vi "Read ModuleA Configuration.vi"(8 "error in (no error)":errorcluster, 11 "ModuleA in":refnum<class "System.lvclass">) -> (0 "error out":errorcluster, 2 "Configuration":T1, 3 "ModuleA out":refnum<class "System.lvclass">)   [LabVIEW 2014, in "System.lvclass"]
uses:
  System.lvclass
  Configuration - cluster.ctl
  <vilib>/JKI/JKI SMO/SMO/SMO.lvclass
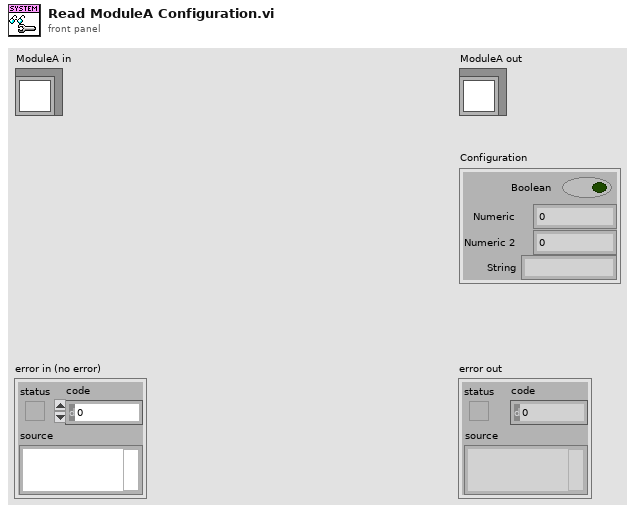
[diagram p1: front panel]
types:
  T1 = typedef "System.lvclass/Configuration - cluster.ctl" = cluster{"Boolean":bool, "Numeric":dbl, "Numeric 2":dbl, "String":string}
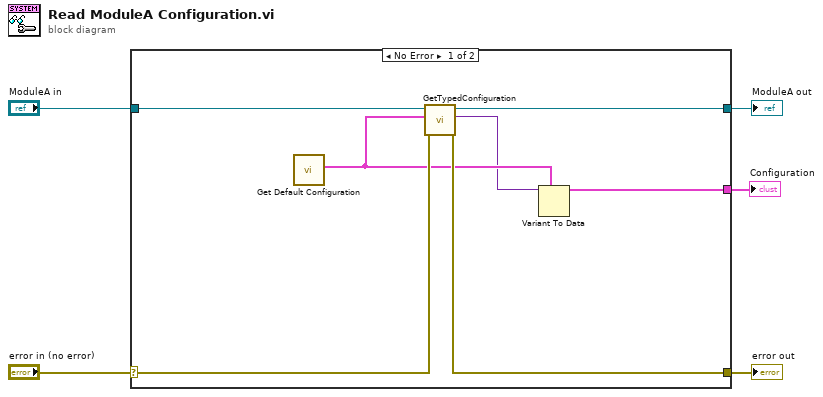
[diagram p0: block diagram]
diagram:
  n1 = case shown="No Error" "error in (no error)" {
    selector: "error in (no error)" -> [w10 w14]
    tunnel: [w9 w14] -> w4
    tunnel: [w11 w13] -> w2
    tunnel: "ModuleA in" -> [w12 w13]
    tunnel: [w6 _] -> w1
    frame No Error {
      n2 = call "Get Default Configuration.vi"() -> ("Configuration"=w8:T1)  [unwired: 11 in]
      n3 = call <vilib>:"GetTypedConfiguration.vi"("error in (no error)"=w10, "Default value"=w8, "SMO"=w12) -> ("error out"=w9:errorcluster, "Variant"=w7:variant, "SMO out"=w11:refnum<class "System.lvclass">)  [unwired: 4 in, 2 out]
      n4 = Variant To Data(type=w8, Variant=w7) -> (data=w6:T1)  [unwired: 1 in, 1 out]
    }
    frame Error {
    }
  }
  "error out" <- w4
  "ModuleA out" <- w2
  "Configuration" <- w1
